vi "StartSnap.vi"(8 "error in (no error)":errorcluster, 11 "Config In":T1 {"Hardware Configuration"."Lasers Configuration"."SettingValues"."785 Power" format="%.1f"; "Hardware Configuration"."Lasers Configuration"."SettingValues"."647 Power" format="%.1f"; "Hardware Configuration"."Lasers Configuration"."SettingValues"."561 Power" format="%.1f"; "Hardware Configuration"."Lasers Configuration"."SettingValues"."532 Power" format="%.1f"; "Hardware Configuration"."Lasers Configuration"."SettingValues"."488 Power" format="%.1f"; "Hardware Configuration"."Lasers Configuration"."SettingValues"."405 Power" format="%.1f"}) -> (0 "error out":errorcluster, 3 "Config Out":T1 {"Hardware Configuration"."Lasers Configuration"."SettingValues"."785 Power" format="%.1f"; "Hardware Configuration"."Lasers Configuration"."SettingValues"."647 Power" format="%.1f"; "Hardware Configuration"."Lasers Configuration"."SettingValues"."561 Power" format="%.1f"; "Hardware Configuration"."Lasers Configuration"."SettingValues"."532 Power" format="%.1f"; "Hardware Configuration"."Lasers Configuration"."SettingValues"."488 Power" format="%.1f"; "Hardware Configuration"."Lasers Configuration"."SettingValues"."405 Power" format="%.1f"})   [LabVIEW 2019]
uses:
  Settings/Settings.ctl
  Support/Hardware Configuration.ctl
  Support/Camera Configuration.ctl
  D:/SDK/PMQI-LabViewSamples/Examples/Dependencies/PVCamNET.dll
  <vilib>/userdefined/High Color/IMAQdx.ctl
  E:/DevHardSoftware/MMicroscopy/HardwareAdapter/Lasers/Dependencies/Oxxius_Boxx.dll
  Lasers/Dependencies/Oxxius_Boxx.dll
  Logging/Logging Configuration.ctl
  controls/UI Configuration.ctl
  controls/CallBack Refs.ctl
  Global.vi
  Logging/Logging.lvlib
  Settings/Settings.lvlib
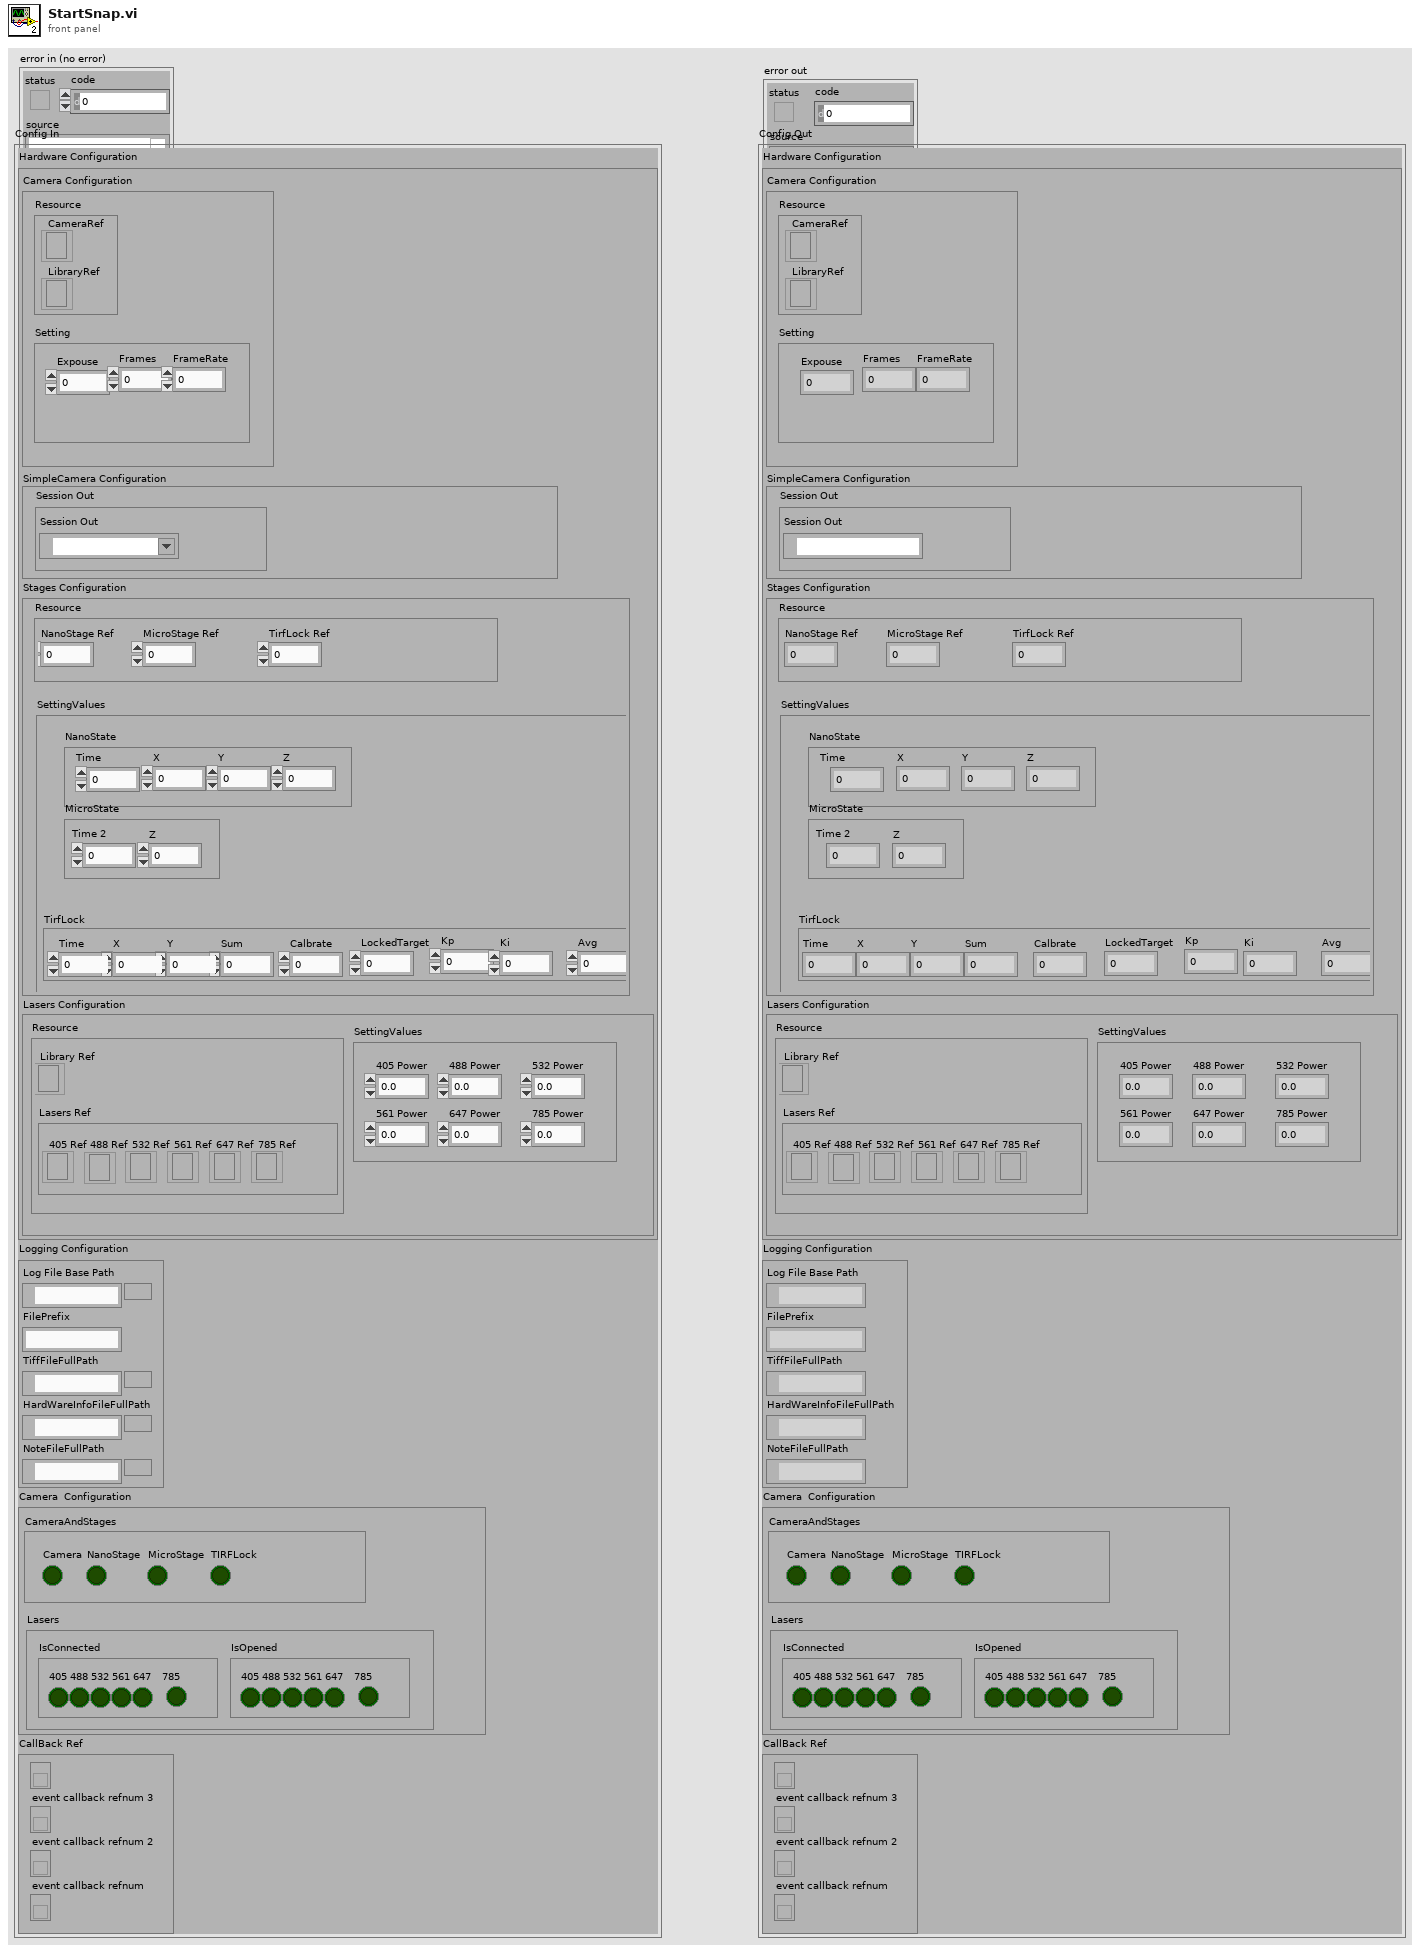
[diagram p1: front panel]
types:
  T1 = typedef "Settings.lvlib/Settings.ctl" = cluster{"Hardware Configuration":T2, "Logging Configuration":T5, "HardWare Status":cluster{"CameraAndStages":T6, "Lasers":cluster{"IsConnected":cluster{"405":bool, "488":bool, "532":bool, "561":bool, "647":bool, "785":bool}, "IsOpened":cluster{"405":bool, "488":bool, "532":bool, "561":bool, "647":bool, "785":bool}}}, "CallBack Ref":T7}
  T2 = typedef "Hardware Configuration.ctl" = cluster{"Camera Configuration":T3, "SimpleCamera Configuration":cluster{"Resource":cluster{"Session Out":T4}}, "Stages Configuration":cluster{"Resource":cluster{"NanoStage Ref":i32, "MicroStage Ref":i32, "TirfLock Ref":i32}, "SettingValues":cluster{"NanoState":cluster{"Time":dbl, "X":dbl, "Y":dbl, "Z":dbl}, "MicroState":cluster{"Time 2":dbl, "Z":dbl}, "TirfLock":cluster{"Time":dbl, "X":dbl, "Y":dbl, "Sum":dbl, "Calbrate":dbl, "LockedTarget":dbl, "Kp":dbl, "Ki":dbl, "Avg":dbl}}}, "Lasers Configuration":cluster{"SettingValues":cluster{"405 Power":sgl, "488 Power":sgl, "532 Power":sgl, "561 Power":sgl, "647 Power":sgl, "785 Power":sgl}, "Resource":cluster{"Library Ref":refnum<k24>, "Lasers Ref":cluster{"405 Ref":refnum<k24>, "488 Ref":refnum<k24>, "532 Ref":refnum<k24>, "561 Ref":refnum<k24>, "647 Ref":refnum<k24>, "785 Ref":refnum<k24>}}}}
  T3 = typedef "Camera Configuration.ctl" = cluster{"Resource":cluster{"CameraRef":refnum<k24>, "LibraryRef":refnum<k24>}, "Setting":cluster{"Expouse":dbl, "Frames":dbl, "FrameRate":dbl}}
  T4 = typedef "IMAQdx.ctl" = refnum<k21>
  T5 = typedef "Logging.lvlib/Logging Configuration.ctl" = cluster{"Log File Base Path":path, "FilePrefix":string, "TiffFileFullPath":path, "HardWareInfoFileFullPath":path, "NoteFileFullPath":path}
  T6 = typedef "UI Configuration.ctl" = cluster{"Camera":bool, "NanoStage":bool, "MicroStage":bool, "TIRFLock":bool}
  T7 = typedef "CallBack Refs.ctl" = cluster{"event callback refnum":refnum<k27>, "event callback refnum 2":refnum<k27>, "event callback refnum 3":refnum<k27>, "event callback refnum 4":refnum<k27>}
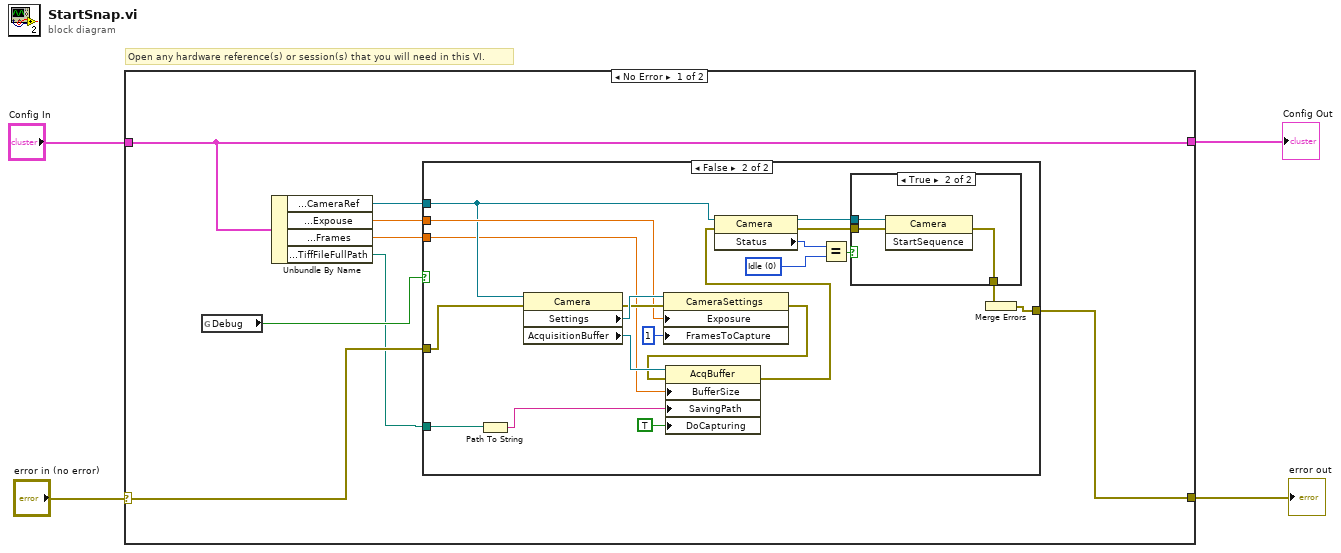
[diagram p0: block diagram]
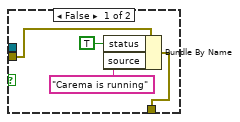
[diagram p3: hidden frame]
diagram:
  # "Open any hardware reference(s) or session(s) that you will need in this VI."
  n1 = case shown="No Error" "error in (no error)" {
    selector: "error in (no error)" -> [w11 w41]
    tunnel: [w10 w41] -> w3
    tunnel: "Config In" -> [w12 w42]
    tunnel: [w12 w42] -> w1
    frame No Error {
      n2 = global read "Global.vi" "Debug"() -> (w9:bool)
      n3 = Unbundle By Name(w12) -> ("Hardware Configuration.Camera Configuration.Resource.CameraRef"=w6:refnum<k24>, "Hardware Configuration.Camera Configuration.Setting.Expouse"=w8:dbl, "Hardware Configuration.Camera Configuration.Setting.Frames"=w7:dbl, "Logging Configuration.TiffFileFullPath"=w5:path)
      n4 = case shown="False" w9 {
        tunnel: w11 -> [w13 w27]
        tunnel: [w13 w29] -> w10
        tunnel: w6 -> [_ w26]
        tunnel: w8 -> [_ w30]
        tunnel: w7 -> [_ w20]
        tunnel: w5 -> [_ w17]
        frame True {
        }
        frame False {
          w25 = 0 items=["Idle", "Capturing"] ("Status")
          n5 = Path To String(path=w17) -> (string=w16:string)
          n6 = property class="Camera"(reference=w26, error in=w27) -> (error out=w32:errorcluster, "Settings"=w33:refnum<k24>, "AcquisitionBuffer"=w31:refnum<k24>)  [unwired: 1 out]
          n7 = property class="CameraSettings"(reference=w33, error in=w32, "Exposure"=w30, "FramesToCapture"=u16 1) -> (error out=w19:errorcluster)  [unwired: 1 out]
          n8 = property class="AcqBuffer"(reference=w31, error in=w19, "BufferSize"=w20, "SavingPath"=w16, "DoCapturing"=TRUE) -> (error out=w18:errorcluster)  [unwired: 1 out]
          n9 = property class="Camera"(reference=w26, error in=w18) -> (reference out=w22:refnum<k24>, error out=w21:errorcluster, "Status"=w24:i32)
          n10 = Equal?(x=w24, y=w25) -> (x = y?=w23:bool)
          n11 = case shown="True" w23 {
            tunnel: [w34 w40] -> w28
            tunnel: w22 -> [_ w39]
            tunnel: w21 -> [w35 w38]
            frame False {
              n12 = Bundle By Name(cluster=w35, "status"=TRUE, "source"="Carema is running") -> (w34:errorcluster)
            }
            frame True {
              n13 = invoke class="Camera" method="StartSequence"(reference=w39, error in=w38) -> (error out=w40:errorcluster)  [unwired: 1 in, 2 out]
            }
          }
          n14 = Merge Errors(w28) -> (w29:errorcluster)
        }
      }
    }
    frame Error {
    }
  }
  "error out" <- w3
  "Config Out" <- w1
